vi "Transmit_Oneshot_Test.vi"() -> ()   [LabVIEW 2014]
uses:
  <vilib>/addons/Modulation/Digital/General/MT Generate Bits (Galois, PN Order).vi
  <vilib>/addons/Modulation/Digital/Support/Common/Validators/mod_Generate Bits Validate.vi
  <vilib>/addons/Modulation/Analog/support/mod_Set Error Source.vi
  <vilib>/addons/Modulation/Digital/Support/Common/Validators/mod_Generate Filter Coefficients Validate.vi
  <vilib>/addons/Modulation/Digital/General/subVIs/mod_Generate Filter Coefficients.vi
  <vilib>/addons/Modulation/Digital/General/MT Generate PSK System Parameters(M).vi
  <vilib>/addons/Modulation/Digital/General/subVIs/mod_Generate Bits PN Sequence.vi
  <vilib>/addons/Modulation/Digital/General/MT Generate PSK Synchronization Parameters (bit array).vi
  <vilib>/addons/Modulation/niDMT.lvlib
panel:
  out "error out":errorcluster
  out "subarray":i8[](array[numeric])
  out "logical AND":bool
  out "output bit stream 2":i8[](array[numeric]) caption="output bit stream"
  out "sync found index (symbols)":dbl format="%.4f"
  out "Constellation Graph":T1(graph) caption="Tx Signal Constellation"
  in  "error in (no error)":errorcluster
  in  "filter parameters":T2={"Alpha"=0.5, "Filter Length"=6, "TX Filter"=enum."Root Raised Cos"} {"Alpha" format="%.2f"}
  in  "USRP IP address":refnum<k15>="192.168.10.1"
  in  "Tx Parameters":T3={"Tx IQ Sampling\nRate [s/sec]"=400000.0, "Tx Frequency [Hz]"=5795000000.0, "Tx Gain [dB]"=0.0, "Tx Antenna"="TX1"} {"Tx Gain [dB]" format="%#.6p"; "Tx Frequency [Hz]" format="%#.6p"; "Tx IQ Sampling\nRate [s/sec]" format="%#.6p"}
  out "Actual Tx Parameters":T3={"Tx IQ Sampling\nRate [s/sec]"=400000.0, "Tx Frequency [Hz]"=915000000.0, "Tx Gain [dB]"=0.0, "Tx Antenna"="TX1"} {"Tx Gain [dB]" format="%#.6p"; "Tx Frequency [Hz]" format="%#.6p"; "Tx IQ Sampling\nRate [s/sec]" format="%#.6p"}
  in  "Custom System Parameters":T4={"Samples per Symbol"=8, "symbol map"=[], "Differential PSK"=enum."disable", "PSK type"=0, "M"=4} caption="M-ary PSK parameters" {"M" min=2 step=2; "PSK type" items=["normal", "shifted", "offset"]; "symbol map" format="%.3f"}
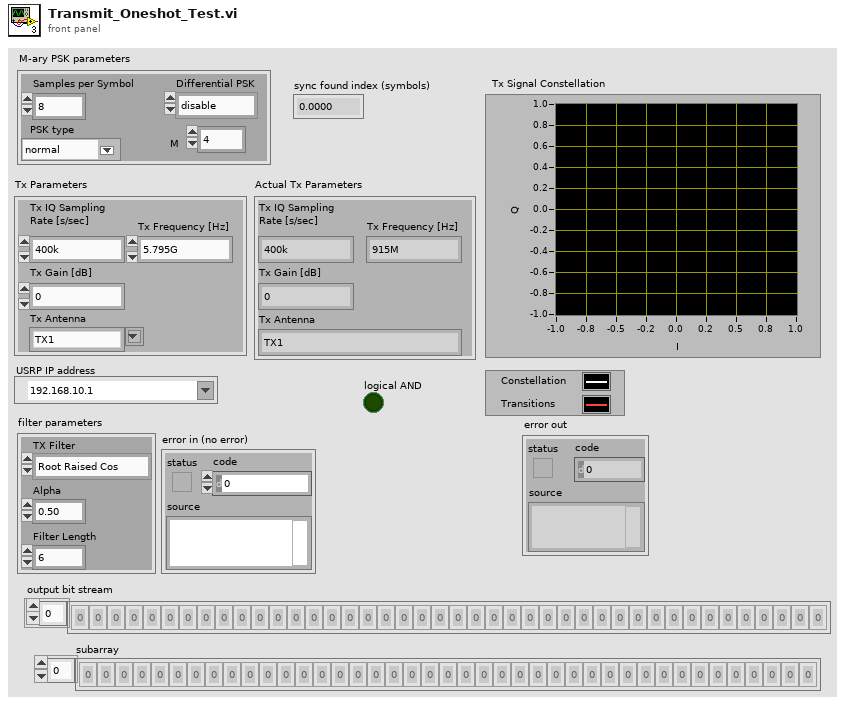
[diagram p1: front panel]
types:
  T1 = cluster{"constellation":dbl[], "oversampled data":dbl[]}[]
  T2 = cluster{"Alpha":dbl, "Filter Length":i32, "TX Filter":enum16{"none", "Raised Cosine", "Root Raised Cos", "Gaussian"}}
  T3 = cluster{"Tx IQ Sampling\nRate [s/sec]":dbl, "Tx Frequency [Hz]":dbl, "Tx Gain [dB]":dbl, "Tx Antenna":string}
  T4 = cluster{"Samples per Symbol":i32, "symbol map":cdb[], "Differential PSK":enum16{"disable", "enable"}, "PSK type":u16, "M":i32}
  T5 = enum16{"FSK", "PSK", "QAM", "MSK", "PAM", "ASK", "CPM"}
  T6 = enum16{"none", "Raised Cosine", "Root Raised Cos", "Gaussian"}
  T7 = cluster{"PSK type":u16, "Samples per Symbol":i32, "Differential PSK":enum16{"disable", "enable"}, "M":i32}
  T8 = typedef "niAMT.lvlib/Complex Data Waveform.ctl" = cluster{"t0":dbl, "dt":dbl, "Y":cdb[]}
  T9 = cluster{"samples per symbol (16)":i32, "symbol map":cdb[], "differential PSK":enum16{"disable", "enable"}, "PSK type":u16}
  T10 = cluster{"expected sync location (symbols)":i32, "sync sequence":cdb[], "sync location uncertainty (symbols)":i32, "sync indent (symbols)":i32}
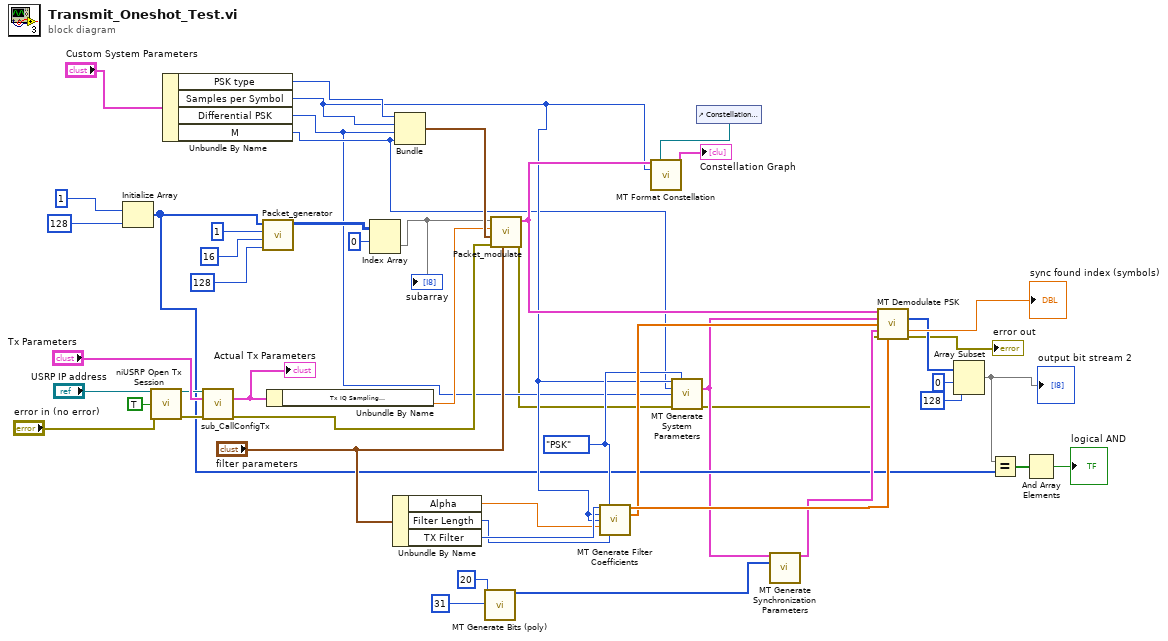
[diagram p0: block diagram]
diagram:
  w10 = T5."PSK" ("modulation type")
  n1 = Initialize Array(i8 1 ("element"), 128 ("dimension size")) -> (w5:i8[])
  n2 = call <instrlib>:"niUSRP Open Tx Session.vi"("device names"="USRP IP address", "reset"=TRUE, "error in (no error)"="error in (no error)") -> ("session handle out"=w37:refnum<k15>, "error out"=w36:errorcluster)  [unwired: 11 in]
  n3 = Unbundle By Name("Custom System Parameters") -> ("PSK type"=w43:u16, "Samples per Symbol"=w8:i32, "Differential PSK"=w6:enum16{"disable", "enable"}, "M"=w7:i32)
  n4 = call "sub_CallConfigTx.vi"("session handle"=w37, "Tx Parameters"="Tx Parameters", "error in"=w36) -> ("Actual Tx Parameters"=w33:T3, "error out"=w30:errorcluster)  [unwired: 10 in, 1 out]
  "Actual Tx Parameters" <- w33
  n5 = call "Packet_generator.vi"("user  bitstream"=w5, "Samples pr burst"=1, "Bits per sample"=16, "Message Bits"=128) -> ("Array"=w41:i8[][])  [unwired: 6 in]
  n6 = Unbundle By Name(w33) -> ("Tx IQ Sampling\nRate [s/sec]"=w31:dbl)
  n7 = Index Array(array=w41, index (row)=0) -> (element=w40:i8[])  [unwired: 1 in]
  "subarray" <- w40
  n8 = Unbundle By Name("filter parameters") -> ("Alpha"=w17:dbl, "Filter Length"=w18:i32, "TX Filter"=w19:T6)
  n9 = Bundle("PSK type"=w43, "Samples per Symbol"=w8, "Differential PSK"=w6, "M"=w7) -> (w42:T7)  [unwired: 1 in]
  n10 = call-poly <vilib>:"MT Generate Bits (poly).vi"("total bits (128)"=20, "PN sequence order (9)"=31) -> ("output bit stream"=w9:i8[])  [unwired: 11 in, 2 out]
  n11 = call "Packet_modulate.vi"("filter parameters"="filter parameters", "error in (no error)"=w30, "PSK Parameters"=w42, "IQ Sampling\nRate [S/sec]"=w31, "input bit stream"=w40) -> ("error out"=w2:errorcluster, "output complex waveform"=w20:T8)  [unwired: 4 in, 1 out]
  n12 = call <vilib>:"MT Generate Filter Coefficients.vi"("pulse shaping filter (none)"=w19, "modulation type"=w10, "pulse shaping samples per symbol (16)"=w8, "matched samples per symbol (16)"=w8, "filter parameter"=w17, "filter length (symbols)"=w18) -> ("pulse shaping filter coefficients"=w15:dbl[], "matched filter coefficients"=w14:dbl[])  [unwired: 7 in, 1 out]
  n13 = call-poly <vilib>:"MT Generate System Parameters.vi"("samples per symbol (16)"=w8, "PSK type"=w10, "M-PSK (4)"=w7, "differential PSK"=w6, "error in (no error)"=w2) -> ("PSK system parameters"=w4:T9, "error out"=w3:errorcluster)  [unwired: 8 in, 1 out]
  n14 = control-ref of="Constellation Graph"() -> (w29:refnum<vi>)
  n15 = call <vilib>:"MT Format Constellation.vi"("waveform"=w20, "constellation reference"=w29, "samples per symbol"=w8) -> ("constellation graph"=→"Constellation Graph":T1)  [unwired: 11 in, 1 out]
  n16 = call-poly <vilib>:"MT Generate Synchronization Parameters.vi"("PSK system parameters"=w4, "sync bits"=w9) -> ("PSK synchronization parameters"=w11:T10)  [unwired: 12 in, 1 out]
  n17 = call <vilib>:"MT Demodulate PSK.vi"("input complex waveform"=w20, "PSK system parameters"=w4, "matched filter coefficients"=w14, "synchronization parameters"=w11, "error in (no error)"=w3, "pulse shaping filter coefficients"=w15) -> ("output bit stream"=w26:i8[], "sync found index (symbols)"=→"sync found index (symbols)":dbl, "error out"=→"error out":errorcluster)  [unwired: 5 in, 2 out]
  n18 = Array Subset(array=w26, index=0, length=128) -> (w23:i8[])
  "output bit stream 2" <- w23
  n19 = Equal?(x=w23, y=w5) -> (x = y?=w22:bool[])
  n20 = And Array Elements(Boolean array=w22) -> (logical AND=→"logical AND":bool)
